vi "Picoammeter - Current Measurement Setup.vi"() -> ()   [LabVIEW 2017]
panel:
  in  "Auto Range":bool
  in  "Delay (Seconds)":dbl
  in  "resource name":string="GPIB0::14::INSTR"
  out "Current Reading":dbl format="%^.2e"
  in  "Current Range":dbl(ring)=0.0001 items=["20mA"=0.02, "2mA"=0.002, "200uA"=0.0002, "20uA"=2e-05, "2uA"=2e-06, "200nA"=2e-07, "20nA"=2e-08, "2nA"=2e-09]
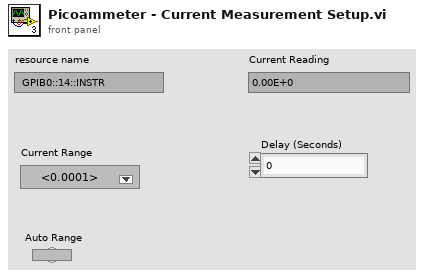
[diagram p1: front panel]
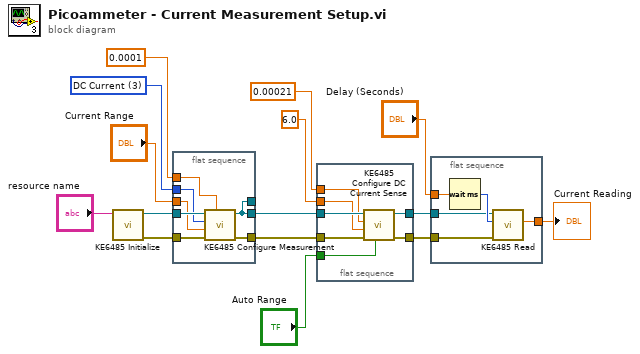
[diagram p0: block diagram]
diagram:
  w10 = 3 items=["DC Volts"=1, "DC Current"=3, "2 Wire Resistance"=5, "Charge"=1004] ("measurement function")
  n1 = call <instrlib>:"KE6485 Initialize.vi"("resource name"="resource name") -> ("error out"=w5:errorcluster, "instrument handle out"=w6:refnum<k15>)  [unwired: 9 in]
  n2 = flat-sequence {
    tunnel: "Current Range" -> [w18]
    tunnel: [w16] -> _
    tunnel: [w22] -> w3
    tunnel: w5 -> [w21]
    tunnel: w6 -> [w20]
    tunnel: w10 -> [w19]
    tunnel: 0.0001 ("resolution (absolute)") -> [w17]
    tunnel: [w16] -> w4
    frame #0 {
      n3 = call <instrlib>:"KE6485 Configure Measurement.vi"("resolution (absolute)"=w17, "error in (no error)"=w21, "range"=w18, "measurement function"=w19, "instrument handle"=w20) -> ("error out"=w22:errorcluster, "instrument handle out"=w16:refnum<k15>)  [unwired: 5 in]
    }
  }
  n4 = flat-sequence {
    tunnel: [w29] -> w2
    tunnel: [w28] -> w1
    tunnel: w4 -> [w26]
    tunnel: w3 -> [w27]
    tunnel: 0.00021 ("range") -> [w25]
    tunnel: 6.0 ("nplc") -> [w24]
    tunnel: "Auto Range" -> [w23]
    frame #0 {
      n5 = call <instrlib>:"KE6485 Configure DC Current Sense.vi"("autorange"=w23, "error in (no error)"=w27, "nplc"=w24, "range"=w25, "instrument handle"=w26) -> ("error out"=w28:errorcluster, "instrument handle out"=w29:refnum<k15>)  [unwired: 5 in]
    }
  }
  n6 = flat-sequence {
    tunnel: [w34] -> w14
    tunnel: "Delay (Seconds)" -> [w32]
    tunnel: w2 -> [w31]
    tunnel: w1 -> [w30]
    frame #0 {
      n7 = Wait (ms)(milliseconds to wait=w32) -> (millisecond timer value=w33:u32)
      n8 = call <instrlib>:"KE6485 Read.vi"("error in (no error)"=w30, "maximum time (ms)"=w33, "instrument handle"=w31) -> ("reading"=w34:dbl)  [unwired: 6 in, 2 out]
    }
  }
  "Current Reading" <- w14
